vi "Test_LogIfError_NoError_ErrorNotLogged.vi"(8 "error in (no error)":errorcluster, 11 "TestCase in":refnum<class "TestComposedLog.lvclass">) -> (0 "error out":errorcluster, 3 "TestCase out":refnum<class "TestComposedLog.lvclass">)   [LabVIEW 2017, in "TestComposedLog.lvclass"]
uses:
  TestComposedLog.lvclass
  Source/Composed Log/Types/Log Level.ctl
  Source/Composed Log/LoggerReference/LoggerReference.lvclass/LoggerReference.ctl
  Source/LVQueue Sink/LVQueue Sink.lvclass/LVQueue Sink.ctl
  e6ba9f54-3038-40c5-af49-aace2fea7c26.vi
  e6ba9f54-3038-40c5-af49-aace2fea7c26.vi/de607bba-af84-4a97-80f8-9ac11e9c77e0.vi
  Source/Composed Log/LoggerReference/Return Aggregate Queues.vi
  Source/Composed Log/LoggerReference/Add Aggregate Log.vi
  e6ba9f54-3038-40c5-af49-aace2fea7c26.vi/de607bba-af84-4a97-80f8-9ac11e9c77e0.vi/89cf1419-8882-47d2-9479-62c2154b8e30.vi
  Source/Composed Log/LoggerReference/Send Add Sink.vi
  Source/LVQueue Sink/LVQueue Sink.lvclass
  C:/CS/Internal/LabVIEW/Logger/Source/Composed Log/Log Sink/Log Sink.lvclass
  Source/Composed Log/Application Logger/Launch Worker Loop.vi
  Source/Composed Log/LoggerReference/Initialize Logger Instance.vi
  Source/Composed Log/Singleton Event Log/Logger Queue FGV.vi
  Source/Composed Log/IErrorFormat/IErrorFormat.lvclass
  Source/Composed Log/LoggerReference/LoggerReference.lvclass
  Source/Composed Log/Log Sink/Log Sink.lvclass
  <vilib>/addons/_JKI Toolkits/VI Tester/TestCase.llb/TestCase.lvclass
  Source/Composed Log/Singleton Event Log/Singleton Event Log.lvlib
  Source/Composed Log/Composed Log.lvlib
  C:/Program Files (x86)/National Instruments/LabVIEW 2017/vi.lib/addons/_JKI Toolkits/VI Tester/TestCase.llb/TestCase.lvclass
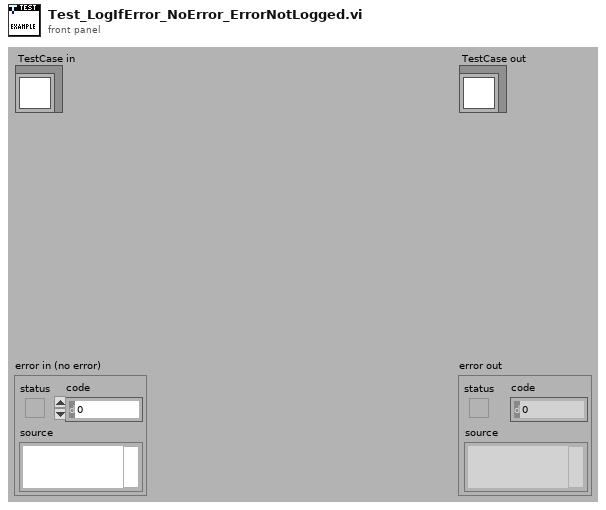
[diagram p1: front panel]
types:
  T1 = typedef "Composed Log.lvlib/Log Level.ctl" = enum16{"Debug", "Info", "Warning", "Error", "Critical"}
  T2 = typedef "Composed Log.lvlib/Log Packet.ctl" = cluster{"Data To Log":string, "Source":string, "Event Level":T1, "Event Time":timestamp}
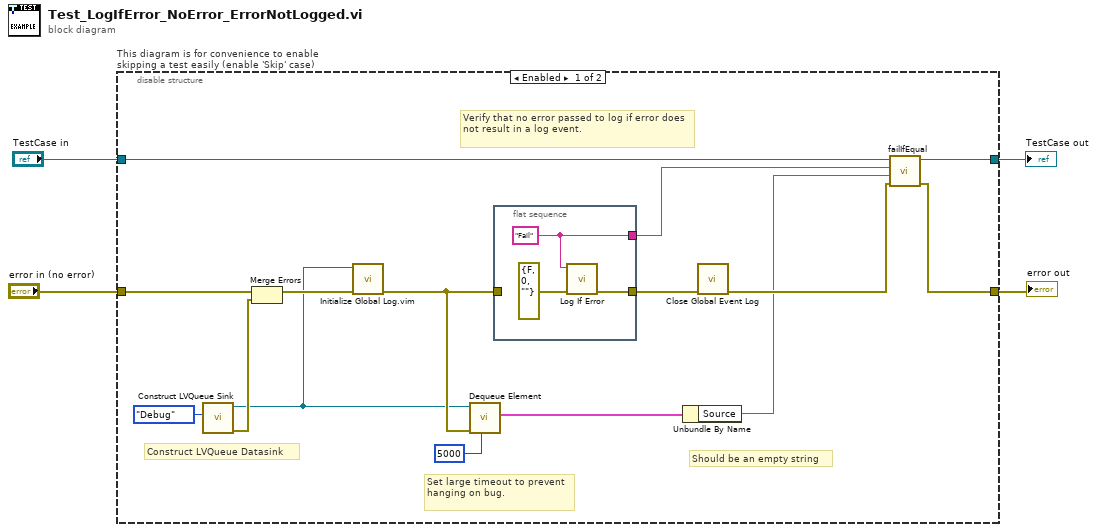
[diagram p0: block diagram]
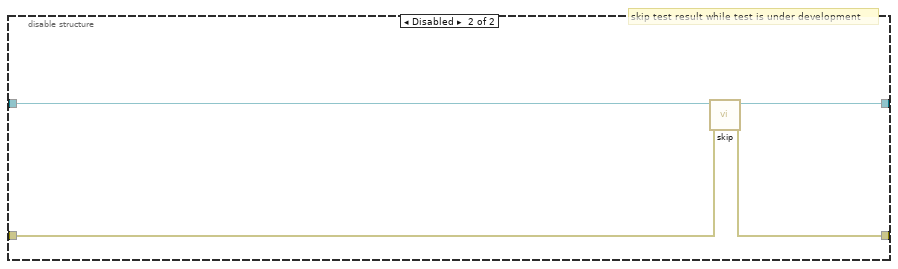
[diagram p2: hidden frame]
diagram:
  n1 = disable-structure "This diagram is for convenience to enable skipping a test easily (enable 'Skip' case)" shown="Enabled" {
    disable-tunnel: "TestCase in" -> [w9 w26]
    disable-tunnel: [w8 w24] -> w1
    disable-tunnel: [w10 w25] -> w3
    disable-tunnel: "error in (no error)" -> [w19 w23]
    frame Enabled {
      # "Should be an empty string"
      # "Construct LVQueue Datasink"
      # "Set large timeout to prevent hanging on bug."
      # "Verify that no error passed to log if error does not result in a log event."
      n2 = call "Construct LVQueue Sink.vi"("LogLevel"=Log_Level."Debug") -> ("error out"=w14:errorcluster, "LVQueue Sink out"=w5:refnum<class "LVQueue Sink.lvclass">)  [unwired: 9 in]
      n3 = Merge Errors(w19, w14) -> (w15:errorcluster)
      n4 = call "Initialize Global Log.vim"("error in (no error)"=w15, "Log Sink(s)"=w5) -> ("error out"=w13:errorcluster)  [unwired: 8 in, 1 out]
      n5 = call "Dequeue Element.vi"("timeout in ms (-1)"=5000, "error in (no error)"=w13, "LVQueue Sink in"=w5) -> ("Log Packet"=w16:T2)  [unwired: 5 in, 3 out]
      n6 = flat-sequence {
        tunnel: w13 -> [_]
        tunnel: [w21] -> w12
        tunnel: [w20] -> w6
        frame #0 {
          w20 = "Fail" ("SourceID")
          n7 = call "Log If Error.vi"("Error In"=errorcluster {"status"=FALSE, "code"=0, "source"=""}, "SourceID"=w20) -> ("error out"=w21:errorcluster)  [unwired: 9 in]
        }
      }
      n8 = Unbundle By Name(w16) -> ("Source"=w7:string)
      n9 = call "Close Global Event Log.vi"("error in (no error)"=w12) -> ("error out"=w11:errorcluster)  [unwired: 10 in]
      n10 = call-dynamic "failIfEqual.vi"("error in (no error)"=w11, "y"=w7, "x"=w6, "TestCase in"=w9) -> ("error out"=w10:errorcluster, "TestCase out"=w8:refnum<class "TestComposedLog.lvclass">)  [unwired: 6 in]
    }
    frame Disabled {
      # "skip test result while test is under development"
      n11 = call <vilib>:"skip.vi"("error in (no error)"=w23, "TestCase in"=w26) -> ("error out"=w25:errorcluster, "TestCase out"=w24:refnum<class "TestComposedLog.lvclass">)  [unwired: 8 in]
    }
  }
  "error out" <- w3
  "TestCase out" <- w1
